vi "Initiate.vi"(8 "error in (no error)":errorcluster, 11 "VISA resource name":refnum<visa-resource-name>) -> (0 "error out":errorcluster, 3 "VISA resource name out":refnum<visa-resource-name>)   [LabVIEW 2017, in "Scope.lvlib" / "Tektronix DPO MSO 2000 4000 Series.lvlib"]
doc: "Initiates a waveform acquisition. An instrument is in an idle state and waits for a trigger after you call this VI.\n\n<B>Note</B>: Use the Initiate VI only with other low-level VIs, such as the Fetch Waveform VI, the Fetch Waveform Measurement VI, and the Abort VI. High-level VIs automatically incorporate the function of the Initiate VI. This VI does not check the status of an instrument."
uses:
  Tektronix DPO MSO 2000 4000 Series.lvlib
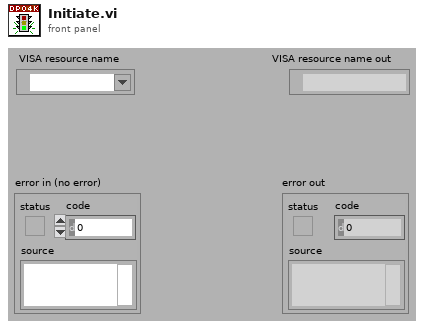
[diagram p1: front panel]
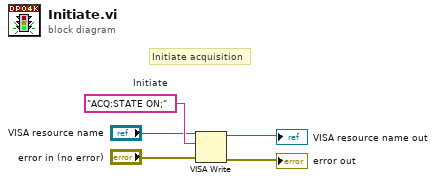
[diagram p0: block diagram]
diagram:
  w5 = "ACQ:STATE ON;"  # Initiate
  # "Initiate acquisition"
  n1 = VISA Write(VISA resource name="VISA resource name", write buffer=w5, error in (no error)="error in (no error)") -> (VISA resource name out=→"VISA resource name out":refnum<visa-resource-name>, error out=→"error out":errorcluster)  [unwired: 1 out]
